vi "pragrama 3.vi"() -> ()   [LabVIEW 2011]
panel:
  out "Observacion":string
  in  "Numero":dbl
  out "Boolean":bool
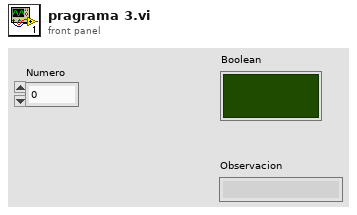
[diagram p1: front panel]
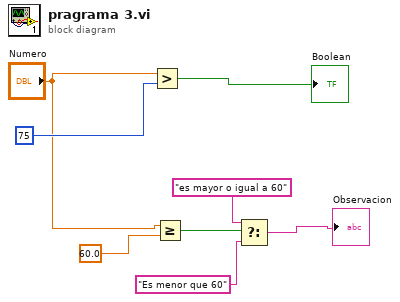
[diagram p0: block diagram]
diagram:
  n1 = Greater?(x="Numero", y=75) -> (0:→"Boolean":bool)
  n2 = Greater Or Equal?(x="Numero", y=60.0) -> (x >= y?=w5:bool)
  n3 = Select(t="es mayor o igual a 60", s=w5, f="Es menor que 60") -> (s? t:f=→"Observacion":string)
